vi "Unflatten.vi"(8 "error in (no error)":errorcluster, 11 "Reader in":refnum<class "Reader.lvclass">) -> (0 "error out":errorcluster, 3 "Reader out":refnum<class "Reader.lvclass">)   [LabVIEW 2017, in "Reader.lvclass"]
uses:
  Reader.lvclass
  Reader.lvclass/Reader.ctl
  Global/File Locations.vi
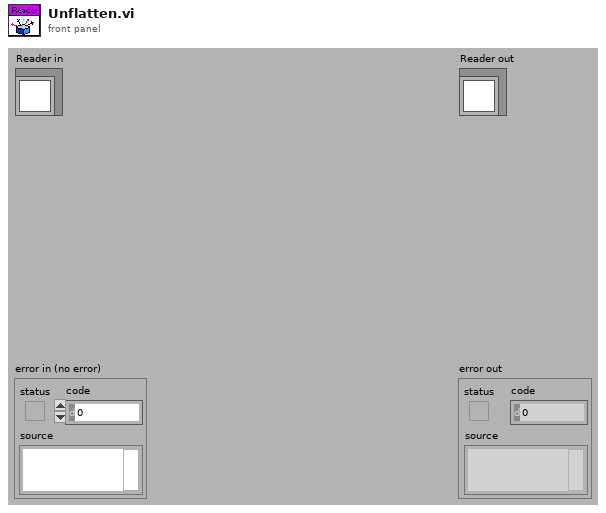
[diagram p1: front panel]
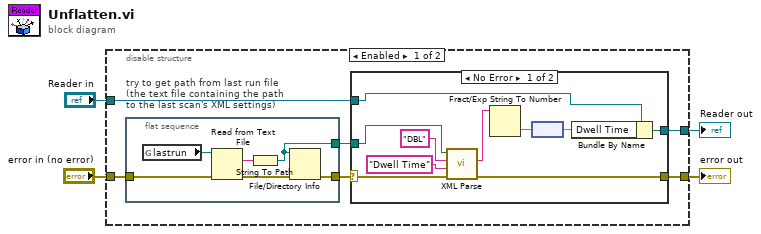
[diagram p0: block diagram]
diagram:
  n1 = disable-structure shown="Enabled" {
    disable-tunnel: [w5 w29] -> w4
    disable-tunnel: "Reader in" -> [w10 w30]
    disable-tunnel: [w9 w30] -> w2
    disable-tunnel: "error in (no error)" -> [w6 w29]
    frame Enabled {
      n2 = flat-sequence "try to get path from last run file\n(the text file containing the path\nto the last scan's XML settings)" {
        tunnel: [w16] -> w8
        tunnel: [w12] -> w7
        tunnel: w6 -> [w11]
        frame #0 {
          n3 = global read "File Locations.vi" "lastrun"() -> (w14:path)
          n4 = Read from Text File(file (use dialog)=w14, error in=w11) -> (text=w15:string, error out=w13:errorcluster)  [unwired: 4 out]
          n5 = String To Path(string=w15) -> (path=w16:path)
          n6 = File/Directory Info(path=w16, error in=w13) -> (error out=w12:errorcluster)  [unwired: 6 out]
        }
      }
      n7 = case shown="No Error" w7 {
        selector: w7 -> [w21 w28]
        tunnel: [w25 w27] -> w9
        tunnel: w10 -> [w26 w27]
        tunnel: w8 -> [w22 _]
        tunnel: [w18 w28] -> w5
        frame No Error {
          n8 = call "XML Parse.vi"("error in (no error)"=w21, "Name String"="Dwell Time", "Type String"="DBL", "Path"=w22) -> ("error out"=w18:errorcluster, "String Out"=w17:string)  [unwired: 6 in]
          n9 = Fract/Exp String To Number(string=w17) -> (number=w24:dbl)  [unwired: 3 in, 1 out]
          n10 = node(w24) -> (w23:dbl[unit])
          n11 = Bundle By Name(cluster=w26, "Dwell Time"=w23) -> (w25:refnum<class "Reader.lvclass">)
        }
        frame Error {
        }
      }
    }
    frame Disabled {
    }
  }
  "error out" <- w4
  "Reader out" <- w2
